vi "Video.vi"() -> ()   [LabVIEW 2018]
doc: "The Grab and Save to AVI VI acquires images continuously using the high-level acquisition VIs, displays them in an image control, and saves the images to an AVI file. A grab is appropriate for high-speed applications that process only one image at a time. Use an AVI file to save multiple images to a single file for post-processing or record images.\n\nIMAQ Init initializes the device. IMAQ Grab Setup initializes the grab function and starts capturing images to an internal software buffer. IMAQ Create creates an image buffer IMAQ Grab Acquire copies the internal buffer to Image out, and an image control displays the image on the front panel. IMAQ Close releases resources associated with the acquisition, and IMAQ Dispose frees the image buffer.\n\nIMAQ AVI Create initializes the AVI file, IMAQ AVI WriteFrame adds each image to the AVI file, and IMAQ AVI Close completes writing to the AVI file. Call IMAQ AVI Create for each AVI file created."
uses:
  <vilib>/userdefined/High Color/IMAQdx.ctl
  <vilib>/vision/driver/NI_Vision_Acquisition_Software.lvlib
  <vilib>/National Instruments/GDrive for LabVIEW/VIs/GDrive.lvlib
panel:
  out "AVI Codecs":string[](array[string])
  out "Processed Frames/s":dbl
  in  "Session In":T1
  in  "Frames Per Second":u32=30
  out "Selected Path":path
  out "Image":T2(plugin-control)
  in  "stop":bool
  # "FPS-ul efectiv"
  # "Playback FPS"
  # "1. Alege Camera"
  # "2. STOP si salveaza videoul"
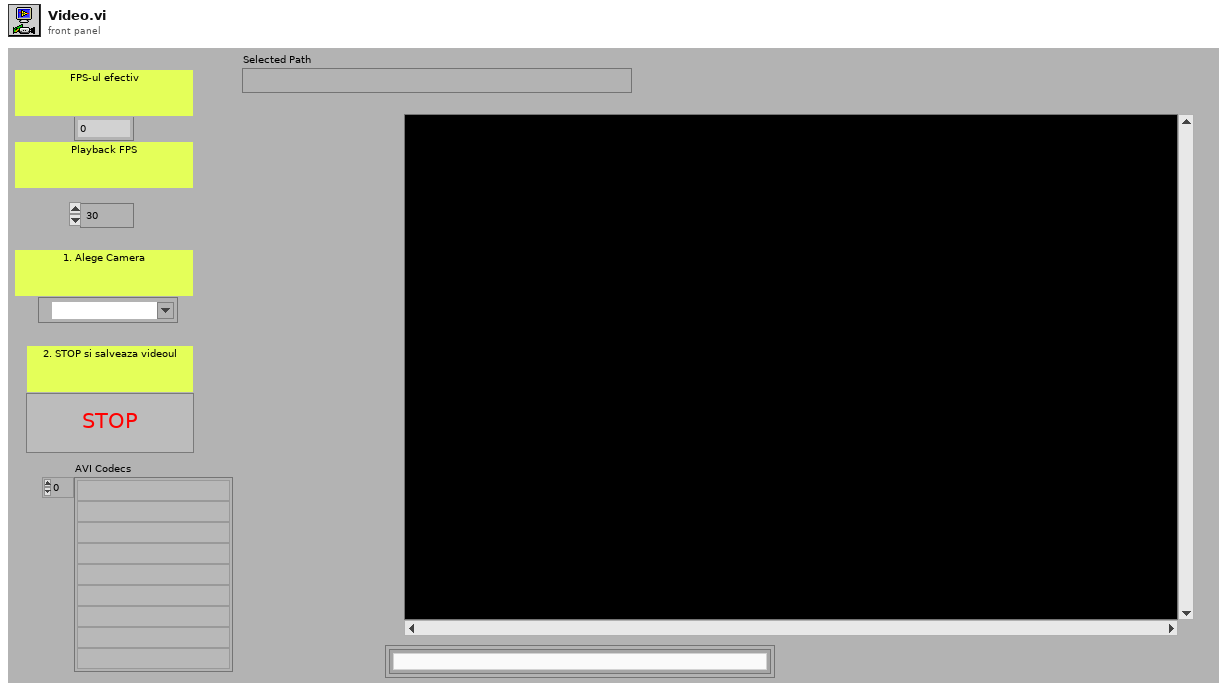
[diagram p1: front panel]
types:
  T1 = typedef "IMAQdx.ctl" = refnum<k21>
  T2 = typedef "IMAQ Image.ctl" = refnum<image>
  T3 = typedef "IMAQ AVI2 Refnum.ctl" = refnum<k20>
  T4 = enum16{"open", "replace", "create", "open or create", "replace or create", "replace or create with confirmation"}
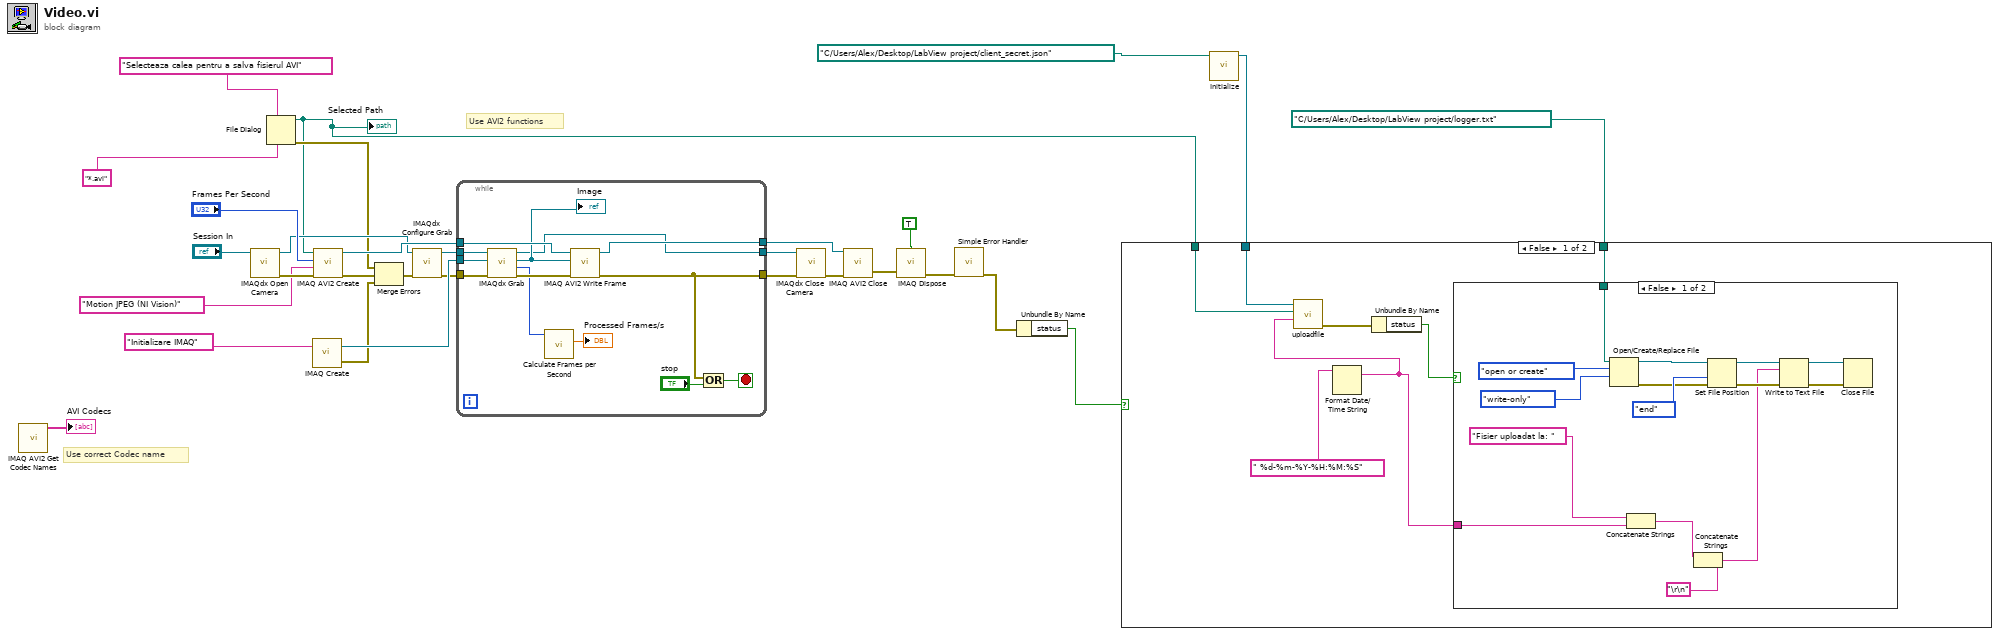
[diagram p0: block diagram]
diagram:
  # "Use correct Codec name"
  # "Use AVI2 functions"
  n1 = call "IMAQ AVI2 Get Codec Names"() -> ("Codec Names"=→"AVI Codecs":string[])  [unwired: 10 in, 1 out]
  n2 = call <vilib>:"IMAQdx Open Camera.vi"("Session In"="Session In") -> ("error out"=w15:errorcluster, "Session Out"=w16:T1)  [unwired: 2 in, 7 out]
  n3 = File Dialog(6:"*.avi" ("pattern"), 7:"Selecteaza calea pentru a salva fisierul AVI" ("prompt")) -> (0:w10:errorcluster, 3:w4:path)  [unwired: 1 in, 6 out]
  "Selected Path" <- w4
  n4 = call "IMAQ Create"("Image Name"="Initializare IMAQ") -> ("New Image"=w30:T2, "error out"=w11:errorcluster)  [unwired: 3 in, 1 out]
  n5 = call "IMAQ AVI2 Create"("error in (no error)"=w15, "Codec"="Motion JPEG (NI Vision)" ("Image Name"), "Frames Per Second"="Frames Per Second", "AVI Path"=w4) -> ("error out"=w26:errorcluster, "AVI Refnum"=w20:T3)  [unwired: 6 in]
  n6 = Merge Errors(w10, w26, w11) -> (w12:errorcluster)
  n7 = call <vilib>:"IMAQdx Configure Grab.vi"("error in"=w12, "Session In"=w16) -> ("error out"=w13:errorcluster, "Session Out"=w17:T1)  [unwired: 1 in, 7 out]
  n8 = while {
    tunnel: [w31] -> w29
    tunnel: w30 -> [w42]
    tunnel: w13 -> [w43]
    tunnel: [w32] -> w28
    tunnel: [w38] -> w25
    tunnel: w20 -> [w37]
    tunnel: w17 -> [w35]
    stop <- w41 stop-if-true
    n9 = call <vilib>:"IMAQdx Grab.vi"("error in"=w43, "Image In"=w42, "Session In"=w35) -> ("error out"=w39:errorcluster, "Buffer Number Out"=w34:u32, "Image Out"=w36:T2, "Session Out"=w31:T1)  [unwired: 1 in, 4 out]
    "Image" <- w36
    n10 = call <vilib>:"Calculate Frames per Second.vi"("Buffer Number"=w34) -> ("Processed Frames/s"=→"Processed Frames/s":dbl)  [unwired: 8 in, 2 out]
    n11 = call "IMAQ AVI2 Write Frame"("error in (no error)"=w39, "Image"=w36, "AVI Refnum"=w37) -> ("error out"=w32:errorcluster, "AVI Refnum (duplicate)"=w38:T3)  [unwired: 6 in, 1 out]
    n12 = Or(x=w32, y="stop") -> (x .or. y?=w41:bool)
  }
  n13 = call <vilib>:"IMAQdx Close Camera.vi"("error in"=w28, "Session In"=w29) -> ("error out"=w23:errorcluster)  [unwired: 9 out]
  n14 = call "IMAQ AVI2 Close"("error in (no error)"=w23, "AVI Refnum"=w25) -> ("error out"=w22:errorcluster)  [unwired: 9 in]
  n15 = call "IMAQ Dispose"("All Images? (No)"=TRUE, "error in (no error)"=w22) -> ("error out"=w24:errorcluster)  [unwired: 1 in, 3 out]
  n16 = call <vilib>:"Simple Error Handler.vi"("error in (no error)"=w24) -> ("error out"=w7:errorcluster)  [unwired: 1 in, 7 out]
  n17 = Unbundle By Name(w7) -> ("status"=w5:bool)
  n18 = call <vilib>:"Initialize.vi"("Path to Secret Client JSON"=path "C:/Users/Alex/Desktop/LabView project/client_secret.json") -> ("Google Drive Service Ref"=w3:refnum<k24>)  [unwired: 9 in, 1 out]
  n19 = case shown="False" w5 {
    tunnel: w4 -> [w46 _]
    tunnel: w3 -> [w45 _]
    tunnel: path "C:/Users/Alex/Desktop/LabView project/logger.txt" ("file path (dialog if empty)") -> [w44 _]
    frame False {
      n20 = Format Date/Time String(time format string (%c)=" %d-%m-%Y-%H:%M:%S") -> (date/time string=w48:string)  [unwired: 2 in]
      n21 = call <vilib>:"uploadfile.vi"("File Name on Drive"=w48, "Local Path"=w46, "Google Drive Service Ref"=w45) -> ("error out"=w49:errorcluster)  [unwired: 7 in]
      n22 = Unbundle By Name(w49) -> ("status"=w47:bool)
      n23 = case shown="False" w47 {
        tunnel: w48 -> [w52 _]
        tunnel: w44 -> [w51 _]
        frame False {
          n24 = Open/Create/Replace File(file path (use dialog)=w51, operation (0:open)=T4."open or create", access (0:read/write)=enum16{"read/write", "read-only", "write-only"}."write-only") -> (refnum out=w62:refnum<file>, error out=w60:errorcluster)  [unwired: 3 in, 1 out]
          n25 = Concatenate Strings("Fisier uploadat la: " ("string"), w52) -> (w55:string)
          n26 = Concatenate Strings(w55, "\r\n") -> (w58:string)
          n27 = Set File Position(refnum=w62, from (0:start)=enum16{"start", "end", "current"}."end", error in=w60) -> (refnum out=w61:refnum<file>, error out=w59:errorcluster)  [unwired: 1 in]
          n28 = Write to Text File(file (use dialog)=w61, text=w58, error in=w59) -> (refnum out=w54:refnum<file>, error out=w53:errorcluster)  [unwired: 1 in, 1 out]
          n29 = Close File(refnum=w54, error in=w53) -> ()  [unwired: 2 out]
        }
        frame True {
        }
      }
    }
    frame True {
    }
  }
